vi "Get Clicked Array Index.vi"(8 "error in":errorcluster, 10 "Coordinates":T1, 11 "CtlRef":refnum<vi>) -> (0 "error out":errorcluster, 1 "Column":i32, 2 "Row":i32)   [LabVIEW 2015]
uses:
  <vilib>/Utility/miscctls.llb/LVPoint32TypeDef.ctl
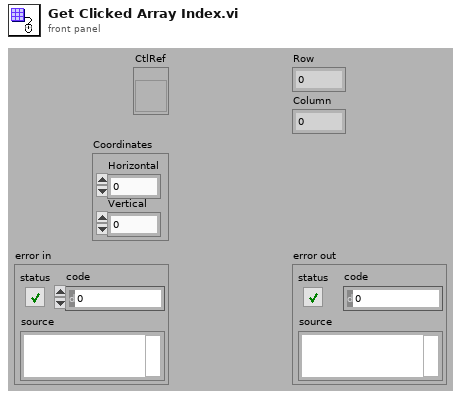
[diagram p1: front panel]
types:
  T1 = typedef "LVPoint32TypeDef.ctl" = cluster{"Horizontal":i32, "Vertical":i32}
  T2 = typedef "LVPositionTypeDef.ctl" = cluster{"Left":i32, "Top":i32}
  T3 = typedef "LVBoundsTypeDef.ctl" = cluster{"Width":u32, "Height":u32}
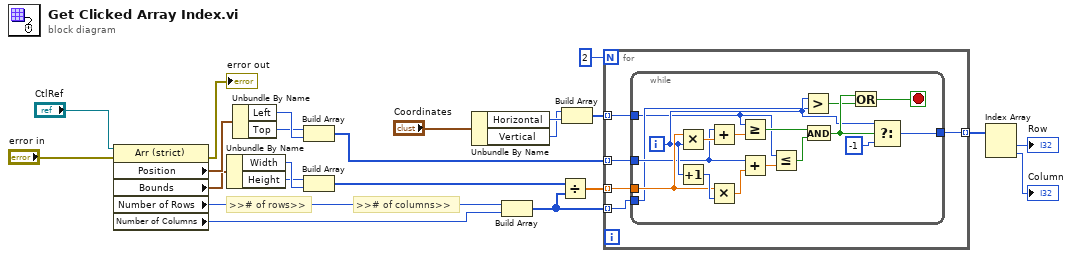
[diagram p0: block diagram]
diagram:
  # ">># of columns>>"
  # ">># of rows>>"
  n1 = property on="Property Node" class="Arr (strict)"(reference="CtlRef", error in="error in") -> (error out=→"error out":errorcluster, "Position"=w23:T2, "Bounds"=w22:T3, "Number of Rows"=w8:u32, "Number of Columns"=w7:u32)  [unwired: 1 out]
  n2 = Unbundle By Name(w22) -> ("Width"=w14:u32, "Height"=w13:u32)
  n3 = Unbundle By Name(w23) -> ("Left"=w16:i32, "Top"=w15:i32)
  n4 = Build Array(w15, w16) -> (w17:i32[])
  n5 = Build Array(w13, w14) -> (w21:u32[])
  n6 = Unbundle By Name("Coordinates") -> ("Horizontal"=w12:i32, "Vertical"=w11:i32)
  n7 = Build Array(w8, w7) -> (w10:u32[])
  n8 = Divide(x=w21, y=w10) -> (x/y=w18:dbl[])
  n9 = Build Array(w11, w12) -> (w19:i32[])
  n10 = for {
    N: 2 -> [_]
    tunnel: w19 -> [w28] mode=indexing
    tunnel: w18 -> [w27] mode=indexing
    tunnel: w17 -> [w26] mode=indexing
    tunnel: [w25] -> w4 mode=indexing
    tunnel: w10 -> [w24] mode=indexing
    n11 = while {
      tunnel: w28 -> [w29]
      tunnel: w27 -> [w35]
      tunnel: w26 -> [w31]
      tunnel: [w40] -> w25
      tunnel: w24 -> [w30]
      i -> [w34]
      stop <- w38 stop-if-true
      n12 = Multiply(x=w35, y=w34) -> (x*y=w32:dbl)
      n13 = Increment(x=w34) -> (x+1=w45:i32)
      n14 = Add(x=w31, y=w32) -> (x+y=w33:dbl)
      n15 = Multiply(x=w35, y=w45) -> (x*y=w43:dbl)
      n16 = Greater Or Equal?(x=w29, y=w33) -> (x >= y?=w42:bool)
      n17 = Add(x=w31, y=w43) -> (x+y=w44:dbl)
      n18 = Less Or Equal?(x=w29, y=w44) -> (x <= y?=w41:bool)
      n19 = Greater?(x=w34, y=w30) -> (0:w36:bool)
      n20 = And(x=w42, y=w41) -> (x .and. y?=w37:bool)
      n21 = Or(x=w37, y=w36) -> (x .or. y?=w38:bool)
      n22 = Select(t=w34, s=w37, f=-1) -> (s? t:f=w40:i32)
    }
  }
  n23 = Index Array(array=w4) -> (element #1=→"Row":i32, element #2=→"Column":i32)  [unwired: 2 in]
